vi "HatchStateControl.vi"(9 "Elevator State":string, 10 "Vacuum Pump Power":dbl) -> ()   [LabVIEW 2018]
uses:
  RobotStates.vi
  Inputs_DriverStation.vi
panel:
  in  "Vacuum Pump Off Time (ms)":u32=1000
  in  "Suction Cup Pulse (ms)":u32=100
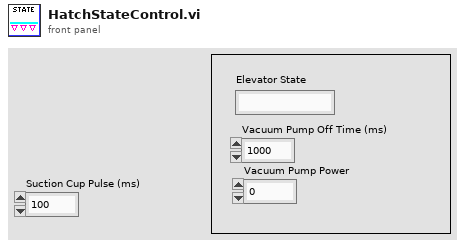
[diagram p1: front panel]
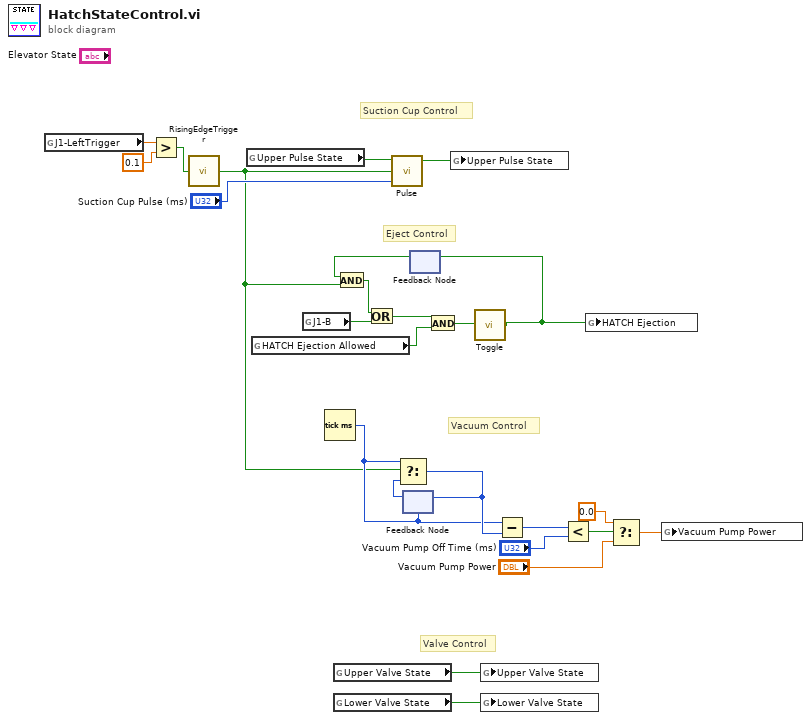
[diagram p0: block diagram]
diagram:
  # "Valve Control"
  # "Eject Control"
  # "Vacuum Control"
  # "Suction Cup Control"
  n1 = global read "Inputs_DriverStation.vi" "J1-LeftTrigger"() -> (w2:dbl)
  n2 = Greater?(x=w2, y=0.1) -> (0:w3:bool)
  n3 = call "RisingEdgeTrigger.vi"("Raw Signal"=w3) -> ("Trigger"=w15:bool)
  n4 = global read "RobotStates.vi" "Upper Pulse State"() -> (w24:bool)
  n5 = global read "RobotStates.vi" "HATCH Ejection Allowed"() -> (w22:bool)
  n6 = global read "Inputs_DriverStation.vi" "J1-B"() -> (w21:bool)
  n7 = Tick Count (ms)() -> (millisecond timer value=w16:u32)
  n8 = global read "RobotStates.vi" "Upper Valve State"() -> (w8:bool)
  n9 = global read "RobotStates.vi" "Lower Valve State"() -> (w7:bool)
  n10 = call "Pulse.vi"("Pulse Duration (ms)"="Suction Cup Pulse (ms)", "Trigger"=w15, "State In"=w24) -> ("State Out"=w23:bool)  [unwired: 2 in]
  n11 = feedback #1(w16) -> (w18:u32)
  n12 = Select(t=w16, s=w15, f=w18) -> (s? t:f=w17:u32)
  n13 = feedback-in #1(w17) -> ()
  n14 = feedback #2() -> (w19:bool)  [unwired: 1 in]
  n15 = And(x=w19, y=w15) -> (x .and. y?=w20:bool)
  n16 = Or(x=w20, y=w21) -> (x .or. y?=w6:bool)
  n17 = And(x=w6, y=w22) -> (x .and. y?=w5:bool)
  n18 = global write "RobotStates.vi" "Upper Pulse State"(w23) -> ()
  n19 = call "Toggle.vi"("Trigger"=w5) -> ("New Mode"=w4:bool)
  n20 = feedback-in #2(w4) -> ()
  n21 = global write "RobotStates.vi" "Upper Valve State"(w8) -> ()
  n22 = global write "RobotStates.vi" "Lower Valve State"(w7) -> ()
  n23 = Subtract(x=w16, y=w17) -> (x-y=w14:u32)
  n24 = Less?(x=w14, y="Vacuum Pump Off Time (ms)") -> (x < y?=w12:bool)
  n25 = global write "RobotStates.vi" "HATCH Ejection"(w4) -> ()
  n26 = Select(t=0.0, s=w12, f="Vacuum Pump Power") -> (s? t:f=w9:dbl)
  n27 = global write "RobotStates.vi" "Vacuum Pump Power"(w9) -> ()
